vi "Next Post Processor Name.vi"(8 "error in (no error)":errorcluster, 11 "Monitor-Pulse in":refnum<class "Monitor-Pulse.lvclass">) -> (0 "error out":errorcluster, 1 "Valid name":bool, 2 "Post processor name":string, 3 "Monitor-Pulse out":refnum<class "Monitor-Pulse.lvclass">)   [LabVIEW 2016, in "Monitor-Pulse.lvclass"]
uses:
  Monitor-Pulse.lvclass
  Monitor-Pulse.lvclass/Monitor-Pulse.ctl
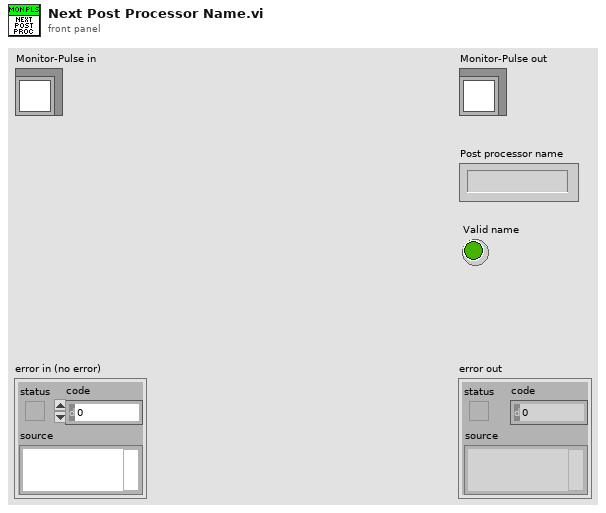
[diagram p1: front panel]
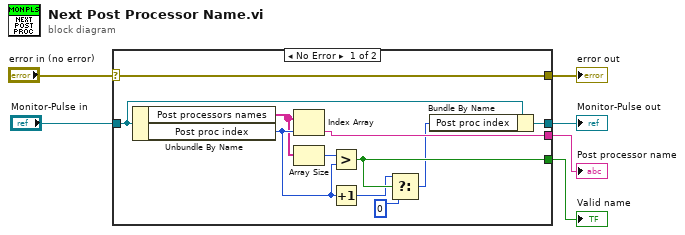
[diagram p0: block diagram]
diagram:
  n1 = case shown="No Error" "error in (no error)" {
    selector: "error in (no error)" -> [w17 w19]
    tunnel: [w17 w19] -> w5
    tunnel: [w12 w18] -> w3
    tunnel: "Monitor-Pulse in" -> [w16 w18]
    tunnel: [w14 _] -> w2
    tunnel: [w10 _] -> w1
    frame No Error {
      n2 = Unbundle By Name(w16) -> ("Post processors names"=w13:string[], "Post proc index"=w15:i32)
      n3 = Index Array(array=w13, index=w15) -> (element=w14:string)
      n4 = Array Size(array=w13) -> (size(s)=w11:i32)
      n5 = Greater?(x=w11, y=w15) -> (0:w10:bool)
      n6 = Increment(x=w15) -> (x+1=w8:i32)
      n7 = Select(t=w8, s=w10, f=0 ("t")) -> (s? t:f=w9:i32)
      n8 = Bundle By Name(cluster=w16, "Post proc index"=w9) -> (w12:refnum<class "Monitor-Pulse.lvclass">)
    }
    frame Error {
    }
  }
  "error out" <- w5
  "Monitor-Pulse out" <- w3
  "Valid name" <- w1
  "Post processor name" <- w2
